vi "LUT - Test destroy DVR.vi"(8 "error in (no error)":errorcluster) -> (0 "error out":errorcluster)   [LabVIEW 2017]
uses:
  <vilib>/addons/_JKI Toolkits/Caraya/classes/Assert/Assert Error.vi
  <vilib>/addons/_JKI Toolkits/Caraya/classes/Test/Test.lvclass
  <vilib>/addons/_JKI Toolkits/Caraya/classes/Assert/Assert.lvclass
  src/LUT/LUT.lvclass
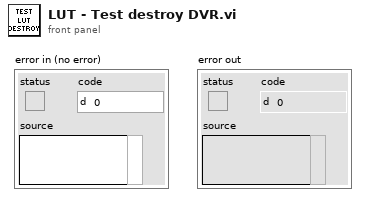
[diagram p1: front panel]
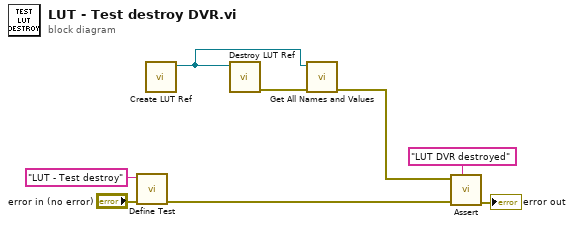
[diagram p0: block diagram]
diagram:
  n1 = call <vilib>:"Define Test.vi"("error in (no error)"="error in (no error)", "Label (VI Title)"="LUT - Test destroy") -> ("error out"=w8:errorcluster)  [unwired: 9 in]
  n2 = call "Create LUT Ref.vi"() -> ("LUT out"=w2:refnum<class "LUT.lvclass">)  [unwired: 10 in, 1 out]
  n3 = call "Destroy LUT Ref.vi"("LUT in"=w2) -> ("error out"=w3:errorcluster)  [unwired: 10 in]
  n4 = call "Get All Names and Values.vi"("error in (no error)"=w3, "LUT in"=w2) -> ("error out"=w1:errorcluster)  [unwired: 6 in, 3 out]
  n5 = call-poly <vilib>:"Assert.vi"("Label"="LUT DVR destroyed", "error in (no error)"=w8, "Error?"=w1) -> ("error out"=→"error out":errorcluster)  [unwired: 8 in]
